vi "Control Panel Controller.vi"(8 "error in":errorcluster) -> ()   [LabVIEW 2019]
doc: "This VI executes continuously carrying out the current operation and responding to updates or new operations. It will often contain the timing or control code that is difficult to place directly in TeleOp. This VI generally opens all sensors and motors and isolates the rest of the robot code from knowing how the operations are carried out."
uses:
  <vilib>/Rock Robotics/WPI/Framework/Completion Status.ctl
  Control Panel Setpoints.ctl
  Control Panel Operations.ctl
  <vilib>/Rock Robotics/SystemInterfaces/i2clib/i2c_bus.ctl
  <vilib>/numeric/Random Number (Range) U64.vi
  <vilib>/numeric/sub_Random U32.vi
  <vilib>/Rock Robotics/Network Tables/NT Write Boolean.vi
panel:
  out "Normalized\nColor":cluster{"R":dbl, "G":dbl, "B":dbl}
  out "Color":u32(colorbox)
  out "Confidence":dbl
  out "Matched Color Name":string
  in  "Interactive Values":T1
  out "Current\nCmd":string
  in  "Buttons":cluster{"Execute Cmd":bool, "Abort Cmd":bool}
  out "Command Timing":cluster{"Start Time (ms)":u32, "Iterations":i32}
  out "Status":T3
  # "Tip: It may be helpful to observe inputs and sensor values.\nYou may also want to display tuning or debugging controls."
  # "Interactive Command: You may fill in the settings for a command\nand schedule it with the Execute button. You can observe and abort\nany command while fine tuning the code for the controller."
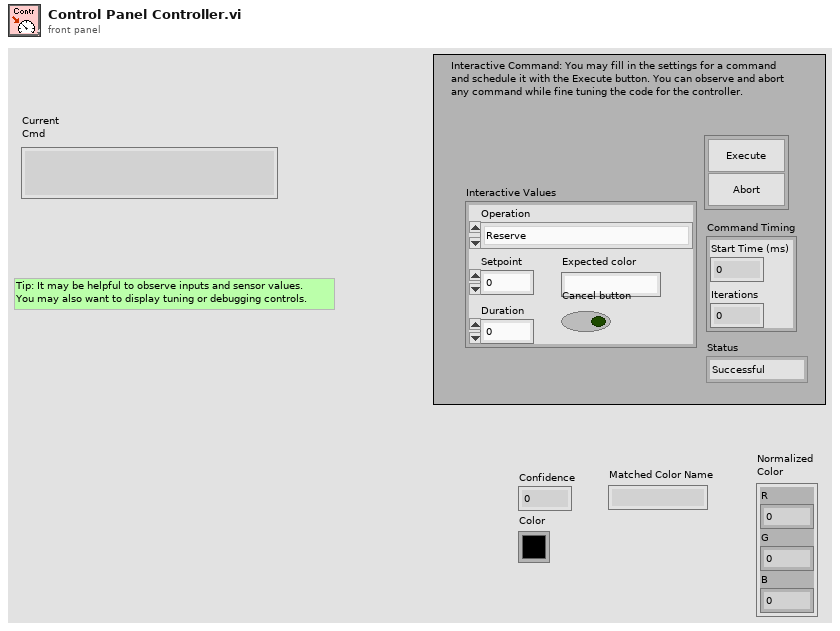
[diagram p1: front panel]
types:
  T1 = typedef "Control Panel Setpoints.ctl" = cluster{"Operation":T2, "Setpoint":dbl, "Duration":dbl, "Expected color":string, "Cancel button":bool}
  T2 = typedef "Control Panel Operations.ctl" = enum16{"Reserve", "RotateRandom", "Read Current", "Immediate", "Rotate", "Rotate to color"}
  T3 = typedef "Completion Status.ctl" = enum16{"Successful", "Aborted", "Incomplete"}
  T4 = typedef "i2c_bus.ctl" = enum16{"I2C On-Board", "I2C MXP", "Invalid"}
  T5 = typedef "Command Status Info.ctl" = cluster{"Name":string, "Status":T3, "notifier out":T6}
  T6 = typedef "Completion Notifier.ctl" = refnum<notifier>
  T7 = cluster{"Current Command":T1, "Command Timing":cluster{"Start Time (ms)":u32, "Iterations":i32}, "Command Arguments":cluster{"Command Info":T5, "Description":string, "Default Command":T1, "queue out":refnum<queue>, "Subsystem Name":string}}
  T8 = typedef "WPI_MotorControlDeviceRef.ctl" = cluster{"DeviceStatus":errorcluster, "Type":T9, "PWM":cluster{"PWM Channel":T10, "DeadBand":T11}, "CAN":cluster{"Device Number":u8, "SetOutput VI Ref":variant, "GetOutput VI Ref":variant, "Enable VI Ref":variant, "Disable VI Ref":variant, "Data":variant}, "Invert":bool, "DIO PWM":cluster{"PWM \"Enable\" Channel":T10, "DIOChannel":T12, "PWM Rate":dbl}}
  T9 = typedef "WPI_MotorControlType.ctl" = enum16{"PWM", "CAN", "DIO PWM"}
  T10 = typedef "FPGA_DIOPWMChannel.ctl" = enum8{"PWM 0", "PWM 1", "PWM 2", "PWM 3", "PWM 4", "PWM 5", "PWM 6", "PWM 7", "PWM 8", "PWM 9", "PWM MXP 0", "PWM MXP 1", "PWM MXP 2", "PWM MXP 3", "PWM MXP 4", "PWM MXP 5", "PWM MXP 6", "PWM MXP 7", "PWM MXP 8", "PWM MXP 9", "Invalid"}
  T11 = typedef "WPI_PWMDeadband.ctl" = cluster{"Name":string, "maxPositivePwm":i32, "minPositivePwm":i32, "centerPwm":i32, "maxNegativePwm":i32, "minNegativePwm":i32, "angularRange":u16}
  T12 = typedef "FPGA_DIOChannel.ctl" = enum8{"DIO 0", "DIO 1", "DIO 2", "DIO 3", "DIO 4", "DIO 5", "DIO 6", "DIO 7", "DIO 8", "DIO 9", "DIO MXP 0", "DIO MXP 1", "DIO MXP 2", "DIO MXP 3", "DIO MXP 4", "DIO MXP 5", "DIO MXP 6", "DIO MXP 7", "DIO MXP 8", "DIO MXP 9", "DIO MXP 10", "DIO MXP 11", "DIO MXP 12", "DIO MXP 13", "DIO MXP 14", "DIO MXP 15", "SPI Port CS1", "SPI Port CS2", "SPI Port CS3", "SPI Port MISO", "SPI Port MOSI", "Invalid"}
  T13 = typedef "Color Sensor V3 DevRef.ctl" = cluster{"I2CDevRef":T14}
  T14 = typedef "WPI_I2CDevRef.ctl" = cluster{"DevStatus":errorcluster, "Device Address":u8, "Handle":i32, "I2C Bus":T4}
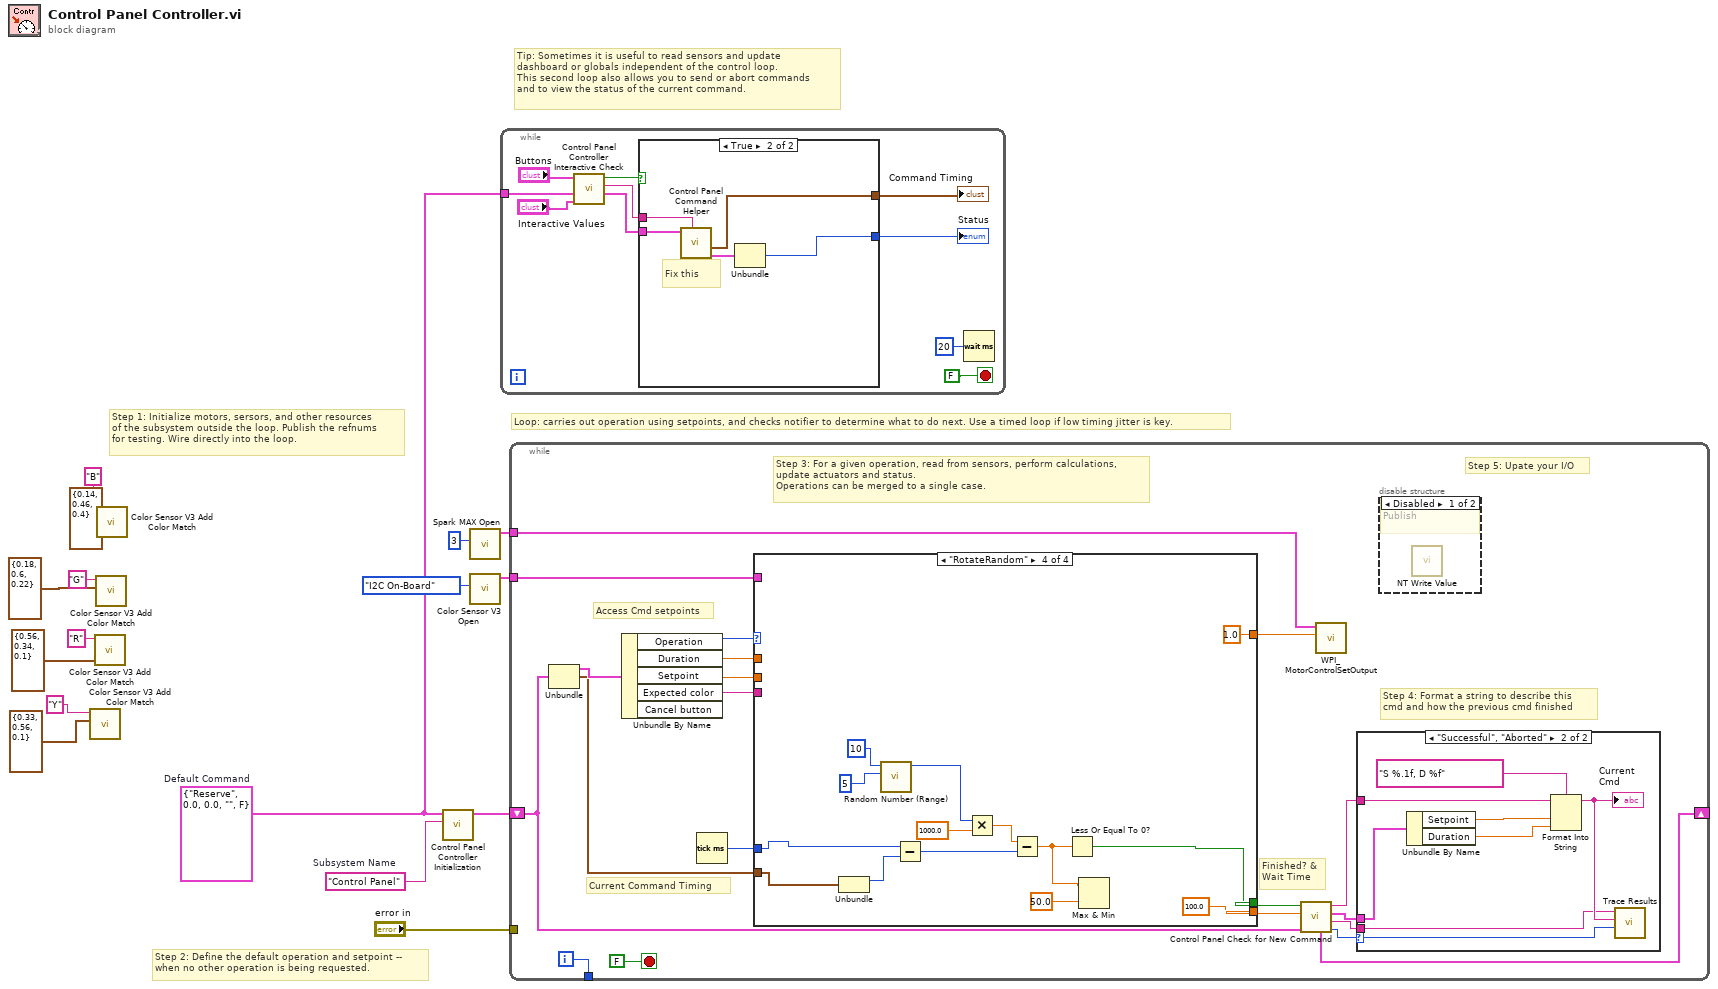
[diagram p0: block diagram]
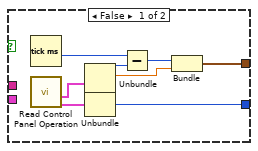
[diagram p2: hidden frame]
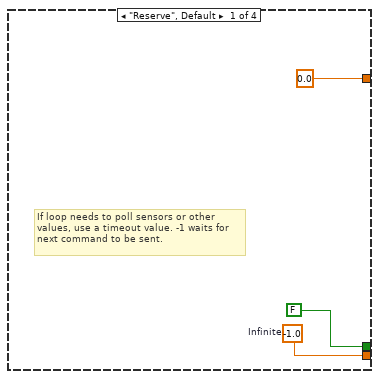
[diagram p5: hidden frame]
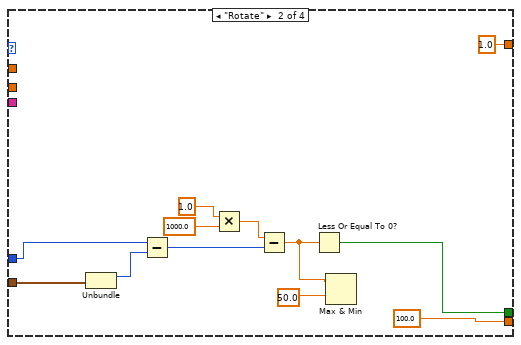
[diagram p6: hidden frame]
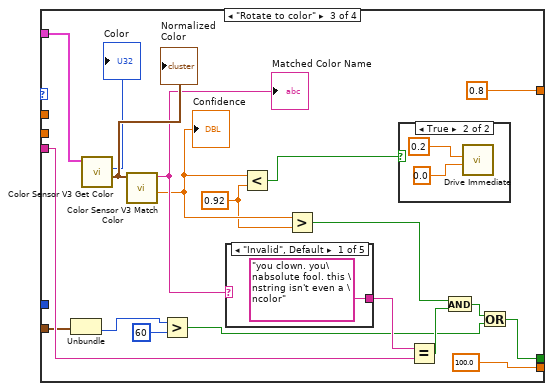
[diagram p7: hidden frame]
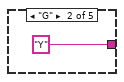
[diagram p8: hidden frame]
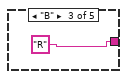
[diagram p9: hidden frame]
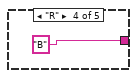
[diagram p10: hidden frame]
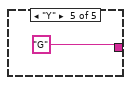
[diagram p11: hidden frame]
diagram:
  w13 = T1 {"Operation"=enum."Reserve", "Setpoint"=0.0, "Duration"=0.0, "Expected color"="", "Cancel button"=FALSE}  # Default Command
  w14 = "Control Panel"  # Subsystem Name
  # "Tip: Sometimes it is useful to read sensors and update\ndashboard or globals independent of the control loop.\nThis second loop also allows you to send or abort commands\nand to view the status of the current command."
  # "Step 2: Define the default operation and setpoint --\nwhen no other operation is being requested."
  # "Step 1: Initialize motors, sersors, and other resources\nof the subsystem outside the loop. Publish the refnums\nfor testing. Wire directly into the loop."
  # "Loop: carries out operation using setpoints, and checks notifier to determine what to do next. Use a timed loop if low timing jitter is key."
  n1 = call <vilib>:"Color Sensor V3 Add Color Match.vi"("Color"=cluster{"R":dbl, "G":dbl, "B":dbl} {"R"=0.33, "G"=0.56, "B"=0.1}, "Name"="Y") -> ()  [unwired: 10 in]
  n2 = call <vilib>:"Color Sensor V3 Add Color Match.vi"("Color"=cluster{"R":dbl, "G":dbl, "B":dbl} {"R"=0.56, "G"=0.34, "B"=0.1}, "Name"="R") -> ()  [unwired: 10 in]
  n3 = call <vilib>:"Color Sensor V3 Add Color Match.vi"("Color"=cluster{"R":dbl, "G":dbl, "B":dbl} {"R"=0.18, "G"=0.6, "B"=0.22}, "Name"="G") -> ()  [unwired: 10 in]
  n4 = call <vilib>:"Color Sensor V3 Add Color Match.vi"("Color"=cluster{"R":dbl, "G":dbl, "B":dbl} {"R"=0.14, "G"=0.46, "B"=0.4}, "Name"="B") -> ()  [unwired: 10 in]
  n5 = call "Control Panel Controller Initialization.vi"("Subsystem Name"=w14, "Default Command"=w13) -> ("Current Command"=w15:T7)  [unwired: 9 in]
  n6 = call <vilib>:"Spark MAX Open.vi"("Device Number"=u8 3) -> ("MotorControlDeviceRef"=w2:T8)  [unwired: 9 in, 1 out]
  n7 = call <vilib>:"Color Sensor V3 Open.vi"("I2C Bus"=i2c_bus."I2C On-Board") -> ("ColorSensorDevRef"=w1:T13)  [unwired: 9 in, 1 out]
  n8 = while {
    tunnel: w13 -> [w23]
    stop <- FALSE stop-if-true
    n9 = call "Control Panel Controller Interactive Check.vi"("Interactive Command in"="Interactive Values", "Default Command"=w23, "Buttons"="Buttons") -> ("Interactive Command out"=w20:T1, "Trace String"=w21:string, "Schedule"=w22:bool)  [unwired: 6 in]
    n10 = case shown="True" w22 {
      tunnel: [w34 w39] -> w19
      tunnel: w20 -> [_ w37]
      tunnel: [w30 w35] -> w18
      tunnel: w21 -> [_ w38]
      frame False {
        n11 = Tick Count (ms)() -> (millisecond timer value=w29:u32)
        n12 = call "Read Control Panel Operation.vi"() -> ("Command Info"=w27:T5, "SubSystem Data"=w28:T1)  [unwired: 9 in, 1 out]
        n13 = Unbundle(w28) -> ("Operation"=w33:T2, "Setpoint"=w31:dbl)  [unwired: 3 out]
        n14 = Unbundle(w27) -> ("Status"=w34:T3)  [unwired: 2 out]
        n15 = Subtract(x=w29, y=w33) -> (x-y=w32:u32)
        n16 = Bundle(w32, "Setpoint"=w31) -> (w30:cluster{u32, "Setpoint":dbl})  [unwired: 1 in]
      }
      frame True {
        # "Fix this"
        n17 = call "Control Panel Command Helper.vi"("Description"=w38, "SubSystem Data"=w37) -> ("Command Info Out"=w36:T5, "Command Timing"=w35:cluster{"Start Time (ms)":u32, "Iterations":i32})  [unwired: 7 in, 1 out]
        n18 = Unbundle(w36) -> ("Status"=w39:T3)  [unwired: 2 out]
      }
    }
    "Status" <- w19
    "Command Timing" <- w18
    n19 = Wait (ms)(milliseconds to wait=u32 20) -> ()  [unwired: 1 out]
  }
  n20 = while {
    shift-right: [w51] -> _
    shift-left: w15 -> [w44]
    tunnel: [w58] -> _
    tunnel: "error in" -> [_]
    tunnel: w2 -> [w42]
    tunnel: w1 -> [w40]
    i -> [w58]
    stop <- FALSE stop-if-true
    # "Step 5: Upate your I/O"
    # "Step 4: Format a string to describe this\ncmd and how the previous cmd finished"
    # "Current Command Timing"
    # "Access Cmd setpoints"
    # "Finished? &\nWait Time"
    # "Step 3: For a given operation, read from sensors, perform calculations,\nupdate actuators and status.\nOperations can be merged to a single case."
    n21 = Unbundle(w44) -> ("Current Command"=w57:T1, "Command Timing"=w53:cluster{"Start Time (ms)":u32, "Iterations":i32})  [unwired: 1 out]
    n22 = Unbundle By Name(w57) -> ("Operation"=w56:T2, "Duration"=w55:dbl, "Setpoint"=w52:dbl, "Expected color"=w43:string)  [unwired: 1 out]
    n23 = Tick Count (ms)() -> (millisecond timer value=w54:u32)
    n24 = case shown="\"RotateRandom\"" w56 {
      tunnel: [w70 100.0 ("Infinite") 100.0 ("Infinite") 100.0 ("Infinite")] -> w49
      tunnel: [FALSE ("ignore previous (F)") w73 w83 w114] -> w50
      tunnel: w53 -> [_ w75 w87 w115]
      tunnel: w55 -> [_ _ _ _]
      tunnel: w54 -> [_ w74 _ w116]
      tunnel: w52 -> [_ _ _ _]
      tunnel: w43 -> [_ _ w93 _]
      tunnel: [0.0 ("Output") 1.0 ("Output") 0.8 ("Output") 1.0 ("Output")] -> w41
      tunnel: w40 -> [_ _ w101 _]
      frame "Reserve", Default {
        w70 = -1.0  # Infinite
        # "If loop needs to poll sensors or other\nvalues, use a timeout value. -1 waits for\nnext command to be sent."
      }
      frame "Rotate" {
        n25 = Unbundle(w75) -> ("Start Time (ms)"=w79:u32)  [unwired: 1 out]
        n26 = Subtract(x=w74, y=w79) -> (x-y=w82:u32)
        n27 = Multiply(x=1.0, y=1000.0) -> (x*y=w81:dbl)
        n28 = Subtract(x=w81, y=w82) -> (x-y=w77:dbl)
        n29 = Less Or Equal To 0?(x=w77) -> (x <= 0?=w73:bool)
        n30 = Max & Min(x=w77, y=50.0) -> ()  [unwired: 2 out]
      }
      frame "Rotate to color" {
        w95 = 0.92 ("y")
        n31 = Unbundle(w87) -> ("Iterations"=w86:i32)  [unwired: 1 out]
        n32 = call <vilib>:"Color Sensor V3 Get Color.vi"("ColorSensorDevRef"=w101) -> ("Normalized Color"=w100:cluster{"R":dbl, "G":dbl, "B":dbl}, "Color"=→"Color":u32)  [unwired: 7 in, 2 out]
        "Normalized\nColor" <- w100
        n33 = call <vilib>:"Color Sensor V3 Match Color.vi"("Measured Color"=w100) -> ("Confidence"=w96:dbl, "Matched Color Name"=w97:string)  [unwired: 8 in, 1 out]
        "Matched Color Name" <- w97
        "Confidence" <- w96
        n34 = Greater?(x=w86, y=u32 60) -> (0:w85:bool)
        n35 = case shown="\"Invalid\", Default" w97 {
          tunnel: ["you clown. you\nabsolute fool. this \nstring isn't even a \ncolor" "Y" "R" "B" "G"] -> w92
          frame "Invalid", Default {
          }
          frame "G" {
          }
          frame "B" {
          }
          frame "R" {
          }
          frame "Y" {
          }
        }
        n36 = Less?(x=w96, y=w95) -> (x < y?=w98:bool)
        n37 = Greater?(x=w96, y=w95) -> (0:w94:bool)
        n38 = case shown="True" w98 {
          frame False {
          }
          frame True {
            n39 = call "Drive Immediate.vi"("Right joystick x"=0.0, "Left joystick y"=0.2) -> ()  [unwired: 9 in, 1 out]
          }
        }
        n40 = Equal?(x=w92, y=w93) -> (x = y?=w91:bool)
        n41 = And(x=w94, y=w91) -> (x .and. y?=w84:bool)
        n42 = Or(x=w84, y=w85) -> (x .or. y?=w83:bool)
      }
      frame "RotateRandom" {
        n43 = Unbundle(w115) -> ("Start Time (ms)"=w118:u32)  [unwired: 1 out]
        n44 = call-poly <vilib>:"Random Number (Range).vi"("lower bound (0)"=u64 5, "upper bound (100)"=u64 10) -> ("number"=w111:u64)  [unwired: 9 in]
        n45 = Subtract(x=w116, y=w118) -> (x-y=w121:u32)
        n46 = Multiply(x=w111, y=1000.0) -> (x*y=w120:dbl)
        n47 = Subtract(x=w120, y=w121) -> (x-y=w117:dbl)
        n48 = Less Or Equal To 0?(x=w117) -> (x <= 0?=w114:bool)
        n49 = Max & Min(x=w117, y=50.0) -> ()  [unwired: 2 out]
      }
    }
    n50 = call "Control Panel Check for New Command.vi"("Current Command"=w44, "Wait time (ms)"=w49, "Finished?"=w50) -> ("Completion"=w45:T3, "Subsystem Name"=w46:string, "Current Command"=w47:T1, "Initial Trace String"=w48:string, "NextCommand"=w51:T7)  [unwired: 4 in]
    n51 = call <vilib>:"WPI_MotorControlSetOutput.vi"("Output"=w41, "MotorControlDevRef"=w42) -> ()  [unwired: 7 in, 3 out]
    n52 = case shown="\"Successful\", \"Aborted\"" w45 {
      selector: w45 -> [_ w67]
      tunnel: w48 -> [_ w63]
      tunnel: w47 -> [_ w64]
      tunnel: w46 -> [_ w60]
      frame "Incomplete", Default {
        # "Continuing current command"
      }
      frame "Successful", "Aborted" {
        # "Report and setup for next command"
        n53 = Unbundle By Name(w64) -> ("Setpoint"=w66:dbl, "Duration"=w61:dbl)
        n54 = Format Into String(format string="S %.1f, D %f", initial string=w63, w66, w61) -> (resulting string=w62:string)  [unwired: 1 in, 1 out]
        "Current\nCmd" <- w62
        n55 = call <vilib>:"Trace Results.vi"("Status of previous command"=w67, "Description"=w62, "Subsystem"=w60) -> ()  [unwired: 9 in]
      }
    }
    n56 = disable-structure shown="Disabled" {
      frame Disabled {
        # "Publish"
        n57 = call-poly <vilib>:"NT Write Value.vi"() -> ()  [unwired: 11 in, 1 out]
      }
      frame Enabled {
      }
    }
  }
